vi "Clear Error.vi"(8 "error in (no error)":errorcluster, 10 "Key":string, 11 "Item Ref in":T1 format="%.0x") -> (0 "error out":errorcluster, 3 "Item Ref out":T1 format="%.0x")   [LabVIEW 2015, in "VeriStand Error API.lvlib"]
doc: "<B>Clear Error</B> looks up the error with the the name <B>Key</B> and removes it from the VeriStand error list."
uses:
  VeriStand Error API.lvlib
  <vilib>/NI Veristand/Custom Device API/Custom Device Item Ref.ctl
  NationalInstruments.VeriStand.SystemStorage
  <vilib>/NI Veristand/Custom Device API/Custom Device API.lvlib
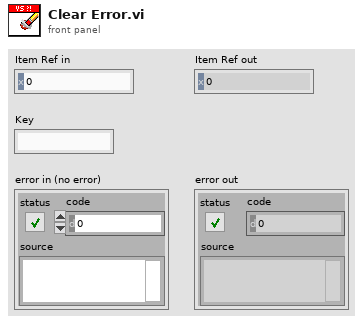
[diagram p1: front panel]
types:
  T1 = typedef "Custom Device API.lvlib/Custom Device Item Ref.ctl" = u64
  T2 = typedef "Custom Device API.lvlib/Custom Device Pointer.ctl" = refnum<k24>
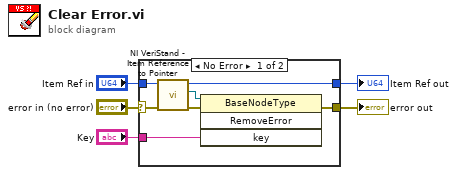
[diagram p0: block diagram]
diagram:
  n1 = case shown="No Error" "error in (no error)" {
    selector: "error in (no error)" -> [w11 w14]
    tunnel: "Item Ref in" -> [w12 w13]
    tunnel: [w9 w13] -> w3
    tunnel: "Key" -> [w8 _]
    tunnel: [w6 w14] -> w1
    frame No Error {
      n2 = call <vilib>:"NI VeriStand - Item Reference to Pointer.vi"("error in (no error)"=w11, "Item Ref in"=w12) -> ("error out"=w7:errorcluster, "Node Pointer"=w10:T2, "Item Ref out"=w9:T1)  [unwired: 6 in, 1 out]
      n3 = invoke class="BaseNodeType" method="RemoveError"(reference=w10, error in=w7, "key"=w8) -> (error out=w6:errorcluster)  [unwired: 1 in, 3 out]
    }
    frame Error {
    }
  }
  "error out" <- w1
  "Item Ref out" <- w3
